vi "determineStiffnessGraphPath.vi"(8 "error in (no error)":errorcluster, 11 "Model in":refnum<class "Model.lvclass">) -> (0 "error out":errorcluster, 2 "graph file path":path, 3 "Model out":refnum<class "Model.lvclass">)   [LabVIEW 2015, in "Model.lvclass"]
uses:
  Model.lvclass
  Model.lvclass/Model.ctl
  <userlib>/Common/Log/Log/Log.lvclass/Log.ctl
  <userlib>/Common/Log/Log/Log.lvclass
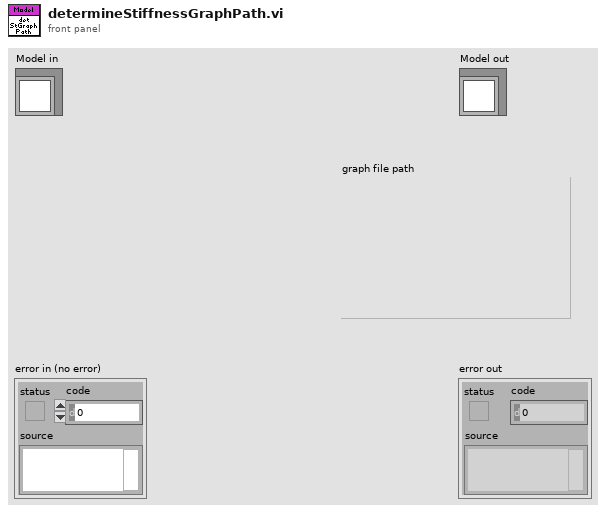
[diagram p1: front panel]
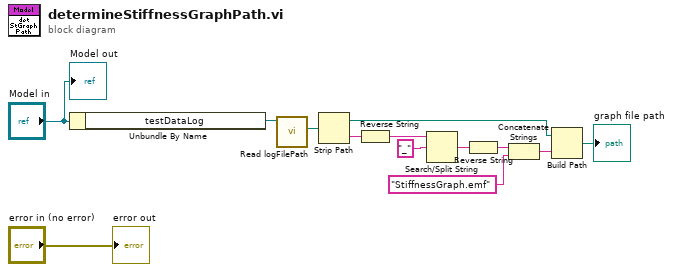
[diagram p0: block diagram]
diagram:
  n1 = Unbundle By Name("Model in") -> ("testDataLog"=w2:refnum<class "TestDataLog.lvclass">)
  n2 = call <userlib>:"Read logFilePath.vi"("Logger in"=w2) -> ("logFilePath"=w1:path)  [unwired: 9 in, 1 out]
  n3 = Strip Path(path=w1) -> (stripped path=w12:path, name=w11:string)
  n4 = Reverse String(1:w11) -> (0:w10:string)
  n5 = Search/Split String(string=w10, search string/char (-)="_") -> (match + rest of string=w8:string)  [unwired: 1 in, 2 out]
  n6 = Reverse String(1:w8) -> (0:w7:string)
  n7 = Concatenate Strings(w7, "StiffnessGraph.emf") -> (w5:string)
  n8 = Build Path(base path=w12, name or relative path=w5) -> (appended path=→"graph file path":path)
  "error out" <- "error in (no error)"
  "Model out" <- "Model in"
